vi "controle de esteira.vi"() -> ()   [LabVIEW 2017]
uses:
  <vilib>/LabVIEW Interface for Arduino/Type Defs/Board Type.ctl
  <vilib>/LabVIEW Interface for Arduino/Type Defs/Connection Type.ctl
  <vilib>/LabVIEW Interface for Arduino/Type Defs/Pin Mode.ctl
  <vilib>/LabVIEW Interface for Arduino/LabVIEW Interface for Arduino.lvlib
panel:
  in  "Habilita":bool
  in  "cx al":bool
  in  "cx md":bool
  out "Desvio":bool
  out "Sopro":bool
  in  "stop":bool
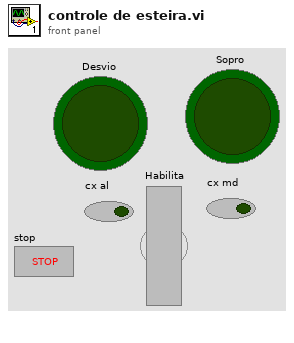
[diagram p1: front panel]
types:
  T1 = typedef "LabVIEW Interface for Arduino.lvlib/Connection Type.ctl" = enum8{"USB / Serial", "XBEE", "BlueSmirf (Bluetooth)"}
  T2 = typedef "LabVIEW Interface for Arduino.lvlib/Board Type.ctl" = enum16{"Uno", "Dimuelanove w/Atmega 328", "Mega 2560"}
  T3 = typedef "LabVIEW Interface for Arduino.lvlib/Arduino Resource.ctl" = cluster{"VISA resource":refnum<visa-resource-name>, "Board Type":T2, "Connection Type":enum8{"USB / Serial"}, "Bytes Per Packet (15)":u8}
  T4 = typedef "LabVIEW Interface for Arduino.lvlib/Pin Mode.ctl" = enum8{"Input", "Output"}
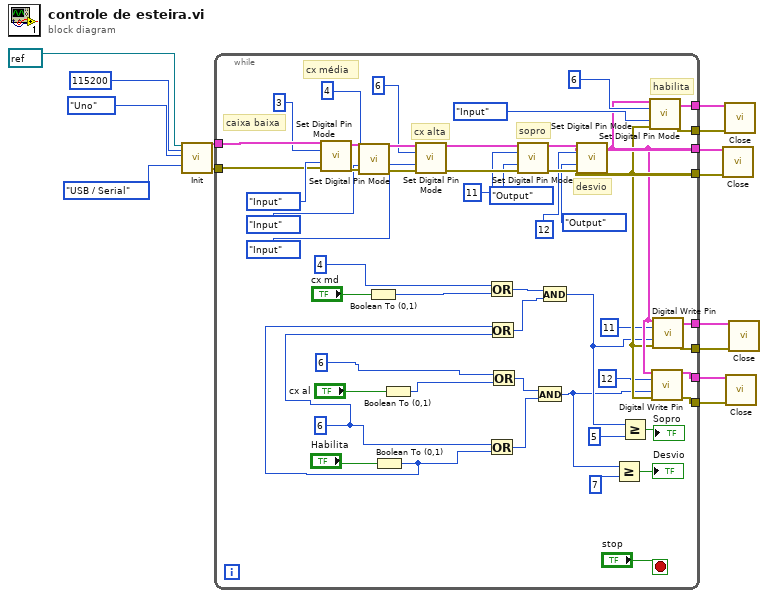
[diagram p0: block diagram]
diagram:
  n1 = call <vilib>:"Init.vi"("VISA resource"=refnum<visa-resource-name> refnum, "Baud Rate (115200)"=u32 115200, "Board Type (Uno)"=Board_Type."Uno", "Connection Type (USB/Serial)"=Connection_Type."USB / Serial") -> ("Arduino Resource"=w10:T3, "error out"=w9:errorcluster)  [unwired: 14 in]
  n2 = while {
    tunnel: w10 -> [w52]
    tunnel: w9 -> [w49]
    tunnel: [w42] -> w8
    tunnel: [w41] -> w7
    tunnel: [w45] -> w6
    tunnel: [w44] -> w5
    tunnel: [w40] -> w4
    tunnel: [w39] -> w3
    tunnel: [w38] -> w2
    tunnel: [w37] -> w1
    stop <- "stop" stop-if-true
    w17 = 6
    # "desvio"
    # "sopro"
    # "habilita"
    # "cx alta"
    # "cx média"
    # "caixa baixa"
    n3 = call <vilib>:"Set Digital Pin Mode.vi"("Arduino Resource"=w52, "Digital I/O Pin"=u8 3, "Pin Mode (Input)"=Pin_Mode."Input", "error in"=w49) -> ("Arduino Resource"=w65:T3, "error out"=w64:errorcluster)  [unwired: 10 in]
    n4 = call <vilib>:"Set Digital Pin Mode.vi"("Arduino Resource"=w65, "Digital I/O Pin"=u8 4, "Pin Mode (Input)"=Pin_Mode."Input", "error in"=w64) -> ("Arduino Resource"=w62:T3, "error out"=w61:errorcluster)  [unwired: 10 in]
    n5 = Boolean To (0,1)(Boolean="cx md") -> (0, 1=w32:i16)
    n6 = Boolean To (0,1)(Boolean="Habilita") -> (0, 1=w16:i16)
    n7 = Boolean To (0,1)(Boolean="cx al") -> (0, 1=w21:i16)
    n8 = call <vilib>:"Set Digital Pin Mode.vi"("Arduino Resource"=w62, "Digital I/O Pin"=u8 6, "Pin Mode (Input)"=Pin_Mode."Input", "error in"=w61) -> ("Arduino Resource"=w59:T3, "error out"=w58:errorcluster)  [unwired: 10 in]
    n9 = Or(x=4, y=w32) -> (x .or. y?=w31:i32)
    n10 = Or(x=w17, y=w16) -> (x .or. y?=w24:i32)
    n11 = Or(x=w16, y=w17) -> (x .or. y?=w15:i32)
    n12 = Or(x=6, y=w21) -> (x .or. y?=w20:i32)
    n13 = call <vilib>:"Set Digital Pin Mode.vi"("Arduino Resource"=w59, "Digital I/O Pin"=11, "Pin Mode (Input)"=Pin_Mode."Output", "error in"=w58) -> ("Arduino Resource"=w56:T3, "error out"=w55:errorcluster)  [unwired: 10 in]
    n14 = And(x=w20, y=w24) -> (x .and. y?=w18:i32)
    n15 = And(x=w31, y=w15) -> (x .and. y?=w28:i32)
    n16 = call <vilib>:"Set Digital Pin Mode.vi"("Arduino Resource"=w56, "Digital I/O Pin"=12, "Pin Mode (Input)"=Pin_Mode."Output", "error in"=w55) -> ("Arduino Resource"=w42:T3, "error out"=w41:errorcluster)  [unwired: 10 in]
    n17 = Greater Or Equal?(x=w18, y=7) -> (x >= y?=→"Desvio":bool)
    n18 = Greater Or Equal?(x=w28, y=5) -> (x >= y?=→"Sopro":bool)
    n19 = call <vilib>:"Set Digital Pin Mode.vi"("Arduino Resource"=w42, "Digital I/O Pin"=u8 6, "Pin Mode (Input)"=Pin_Mode."Input", "error in"=w41) -> ("Arduino Resource"=w45:T3, "error out"=w44:errorcluster)  [unwired: 10 in]
    n20 = call <vilib>:"Digital Write Pin.vi"("Arduino Resource"=w42, "Digital I/O Pin (0)"=u8 12, "Value (0)"=w18, "error in"=w41) -> ("Arduino Resource"=w38:T3, "error out"=w37:errorcluster)  [unwired: 10 in]
    n21 = call <vilib>:"Digital Write Pin.vi"("Arduino Resource"=w42, "Digital I/O Pin (0)"=u8 11, "Value (0)"=w28, "error in"=w41) -> ("Arduino Resource"=w40:T3, "error out"=w39:errorcluster)  [unwired: 10 in]
  }
  n22 = call <vilib>:"Close.vi"("Arduino Resource"=w8, "error in"=w7) -> ()  [unwired: 13 in, 1 out]
  n23 = call <vilib>:"Close.vi"("Arduino Resource"=w6, "error in"=w5) -> ()  [unwired: 13 in, 1 out]
  n24 = call <vilib>:"Close.vi"("Arduino Resource"=w2, "error in"=w1) -> ()  [unwired: 13 in, 1 out]
  n25 = call <vilib>:"Close.vi"("Arduino Resource"=w4, "error in"=w3) -> ()  [unwired: 13 in, 1 out]
